vi "ProdaNG.Init.vi"(7 "DbgLogPath (empty: off)":path, 8 "error in (no error)":errorcluster, 11 "numContexts (0: unlimited)":i32) -> (0 "error out":errorcluster)   [LabVIEW 2016]
doc: "InitProDll must be called from the Main Thread before any other function is used.\nParameter:\nnumContexts is an Integer, which indicates how many parallel logins should be allowed by the DLL later:\n0 means: A Shared Context is being used. This is intended for backward compatibility, because only one connection and context is being used. All operations use this one connection. The usage is secure for Multi-threading.\n>0 means: A new context is being used for every login to the database.\nReturncodes:\n0 No error\n< 0 ORACLE error code\n> 0 Windows error code (errno)"
uses:
  LowLevel/ProdaNG.Global.vi
  prodllNG.dll
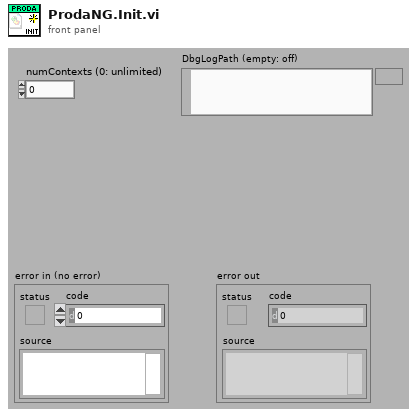
[diagram p1: front panel]
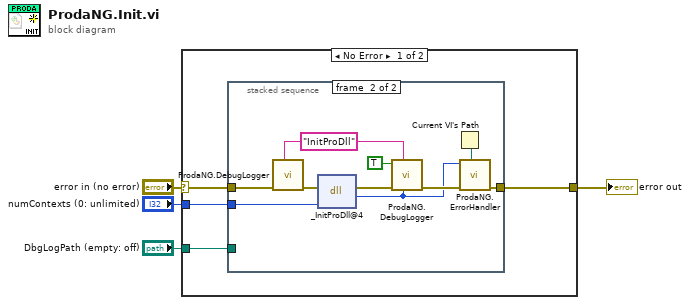
[diagram p0: block diagram]
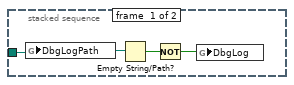
[diagram p2: hidden frame]
diagram:
  n1 = case shown="No Error" "error in (no error)" {
    selector: "error in (no error)" -> [w6 w22]
    tunnel: [w8 w22] -> w3
    tunnel: "numContexts (0: unlimited)" -> [w7 _]
    tunnel: "DbgLogPath (empty: off)" -> [w5 _]
    frame No Error {
      n2 = stacked-sequence {
        tunnel: [_ w21] -> w8
        tunnel: w7 -> [_ w19]
        tunnel: w6 -> [_ w14]
        tunnel: w5 -> [w9 _]
        frame #0 {
          n3 = global write "ProdaNG.Global.vi" "DbgLogPath"(w9) -> ()
          n4 = Empty String/Path?(string/path=w9) -> (empty?=w11:bool)
          n5 = Not(x=w11) -> (.not. x?=w10:bool)
          n6 = global write "ProdaNG.Global.vi" "DbgLog"(w10) -> ()
        }
        frame #1 {
          w13 = "InitProDll" ("cmd")
          n7 = call "ProdaNG.DebugLogger.vi"("cmd"=w13, "error in (no error)"=w14) -> ("error out"=w17:errorcluster)  [unwired: 9 in]
          n8 = dll-call lib="D:/Maszup/WABCO/SVN/LineTraceSystem/SOFTWARE/sources/Database/ProdaNG/prodllNG.dll" fn="_InitProDll@4" ("ProDll.dll:InitProDll")(error in=w17, "numContexts"=w19) -> (error out=w16:errorcluster, "return type"=w12:i32)  [unwired: 3 in, 1 out]
          n9 = call "ProdaNG.DebugLogger.vi"("return type"=w12, "cmd"=w13, "error in (no error)"=w16, "done? (F)"=TRUE) -> ("error out"=w15:errorcluster)  [unwired: 7 in]
          n10 = Current VI's Path() -> (path=w20:path)
          n11 = call "ProdaNG.ErrorHandler.vi"("Path"=w20, "error in"=w15, "output_parameter"=w12) -> ("error out"=w21:errorcluster)  [unwired: 8 in]
        }
      }
    }
    frame Error {
    }
  }
  "error out" <- w3
